vi "Action.vi"() -> ()   [LabVIEW 2014]
uses:
  APIs/Message Queue/WINFAS 2 Message Queue.lvlib
  APIs/Message Queue/Enqueue Message (Array).vi
  APIs/Message Queue/Enqueue Message (Single).vi
  Classes/AutoZero/AutoZero.lvclass
  TypeDefs/STEP State.ctl
  APIs/Message Queue/Message Cluster.ctl
panel:
  in  "CORE":refnum<queue>
  in  "STEP State":T1
  out "AutoZero out":refnum<class "AutoZero.lvclass">
  in  "AutoZero in":refnum<class "AutoZero.lvclass">
  out "error out":errorcluster
  in  "error in (no error)":errorcluster
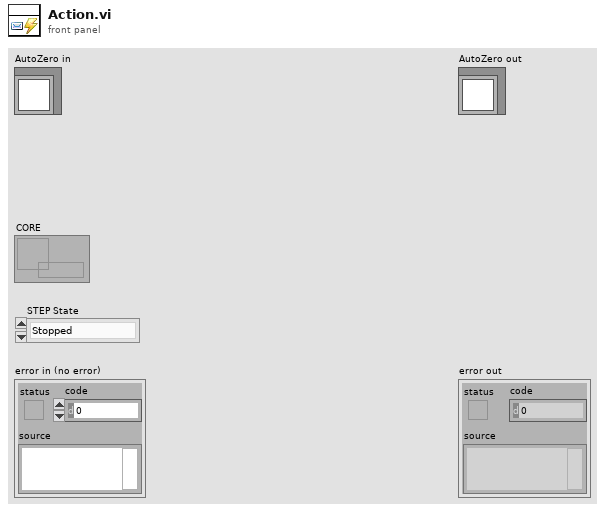
[diagram p1: front panel]
types:
  T1 = typedef "Seq-MathLoop.lvlib/STEP State.ctl" = enum16{"Stopped", "First Call", "Idle...", "Advance OK", "Alarm", "Output Security", "Error"}
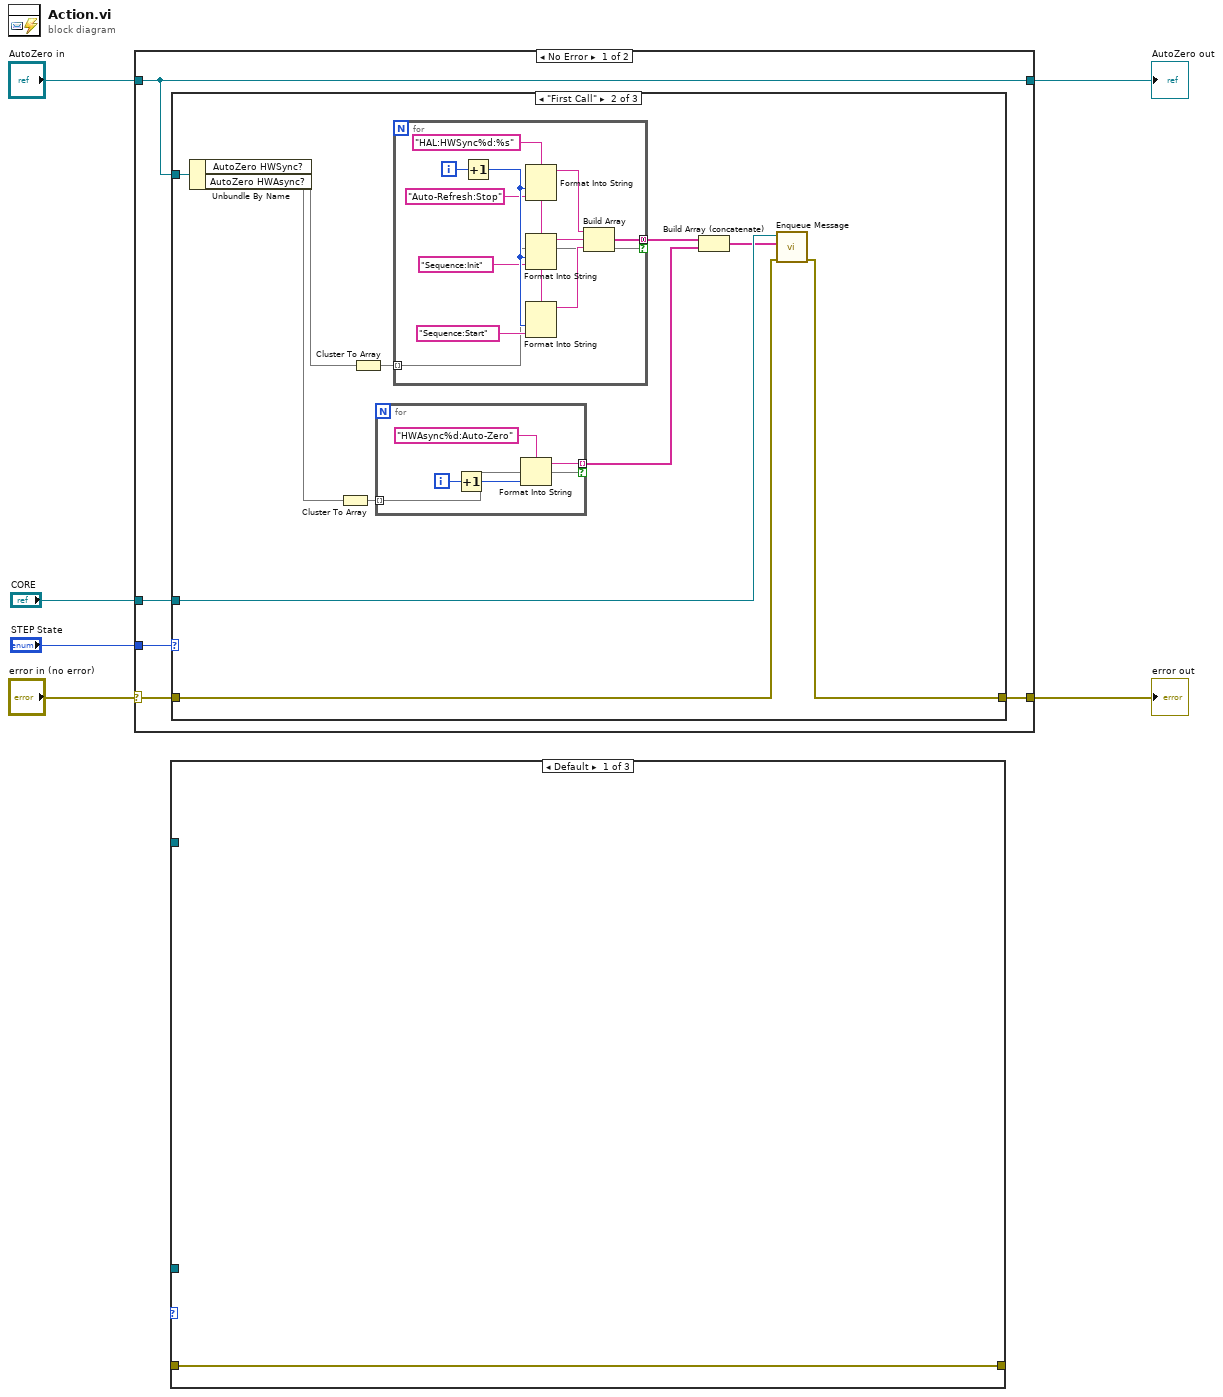
[diagram p0: block diagram]
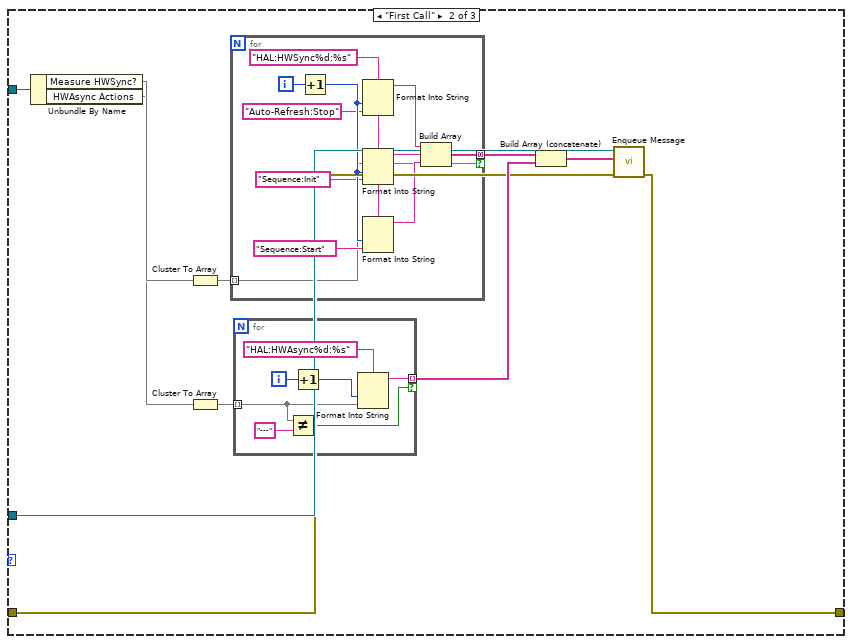
[diagram p2: hidden frame]
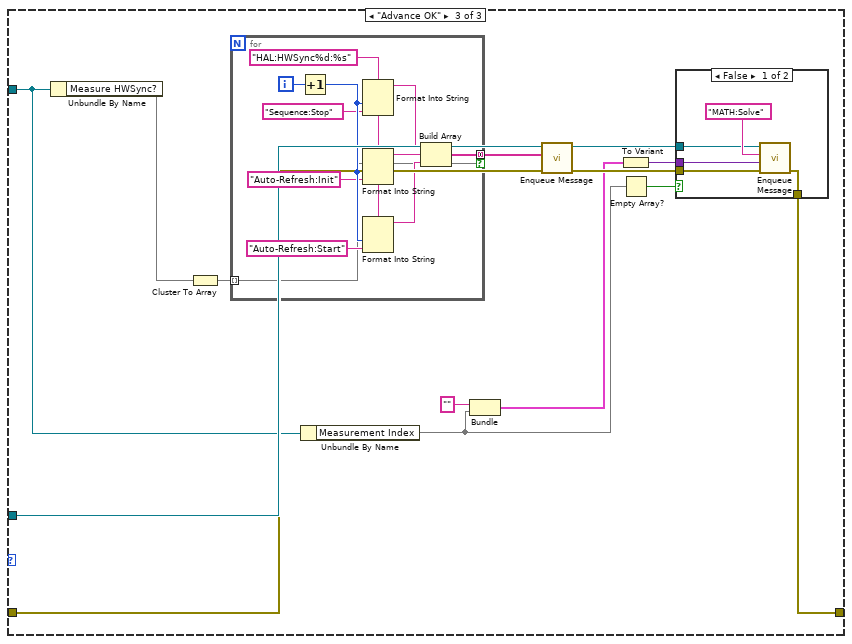
[diagram p3: hidden frame]
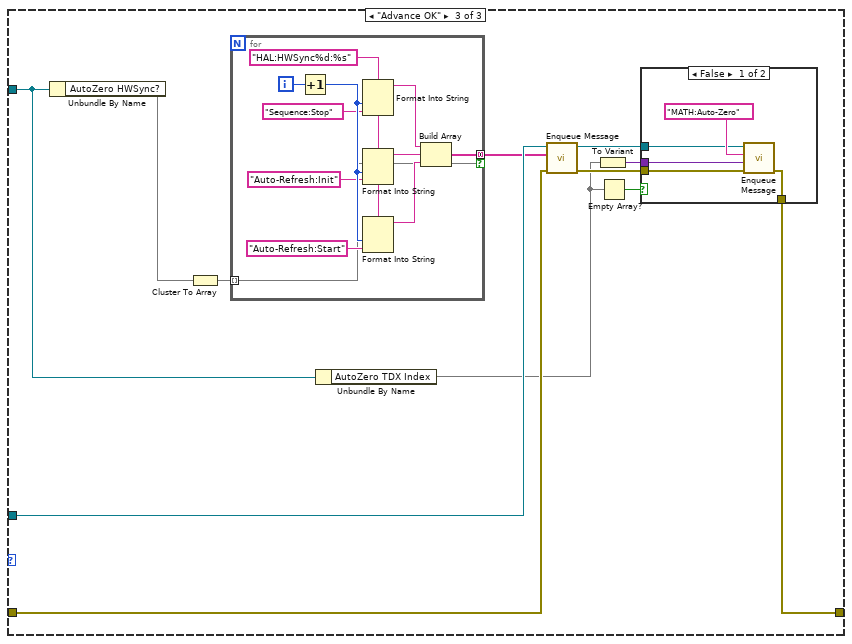
[diagram p6: hidden frame]
diagram:
  n1 = case shown="No Error" "error in (no error)" {
    selector: "error in (no error)" -> [w8 w70]
    tunnel: [w7 w70] -> w3
    tunnel: [w9 w69] -> w5
    tunnel: "AutoZero in" -> [w9 w69]
    tunnel: "CORE" -> [w10 _]
    tunnel: "STEP State" -> [w11 _]
    frame No Error {
      n2 = case shown="\"First Call\"" w11 {
        tunnel: w10 -> [_ w16 w49]
        tunnel: w9 -> [_ w22 w44]
        tunnel: w8 -> [w12 w14 w48]
        tunnel: [w12 w13 w45] -> w7
        frame Default {
        }
        frame "First Call" {
          n3 = Unbundle By Name(w22) -> ("AutoZero HWSync?"=w21, "AutoZero HWAsync?"=w20)
          n4 = Cluster To Array(cluster=w20) -> (array=w19:void[])
          n5 = Cluster To Array(cluster=w21) -> (array=w23:void[])
          n6 = for {
            tunnel: w19 -> [w24] mode=indexing
            tunnel: [w25] -> w17 mode=indexing if=w24
            i -> [w27]
            n7 = Increment(x=w27) -> (x+1=w26:i32)
            n8 = Format Into String(format string="HWAsync%d:Auto-Zero", w26) -> (resulting string=w25:string)  [unwired: 2 in, 1 out]
          }
          n9 = for {
            tunnel: w23 -> [w29] mode=indexing
            tunnel: [w30] -> w18 mode=concatenating if=w29
            i -> [w39]
            w38 = "HAL:HWSync%d:%s" ("format string")
            n10 = Increment(x=w39) -> (x+1=w37:i32)
            n11 = Format Into String(format string=w38, w37, "Auto-Refresh:Stop" ("format string")) -> (resulting string=w33:string)  [unwired: 2 in, 1 out]
            n12 = Format Into String(format string=w38, w37, "Sequence:Init" ("format string")) -> (resulting string=w32:string)  [unwired: 2 in, 1 out]
            n13 = Format Into String(format string=w38, w37, "Sequence:Start" ("format string")) -> (resulting string=w31:string)  [unwired: 2 in, 1 out]
            n14 = Build Array(w33, w32, w31) -> (w30:string[])
          }
          n15 = Build Array (concatenate)(w18, w17) -> (w15:string[])
          n16 = call-poly "Enqueue Message.vi"("error in (no error)"=w14, "Message Array"=w15, "Message Queue"=w16) -> ("error out"=w13:errorcluster)  [unwired: 7 in, 1 out]
        }
        frame "Advance OK" {
          n17 = Unbundle By Name(w44) -> ("AutoZero HWSync?"=w50)
          n18 = Cluster To Array(cluster=w50) -> (array=w51:void[])
          n19 = for {
            tunnel: w51 -> [w58] mode=indexing
            tunnel: [w59] -> w47 mode=concatenating if=w58
            i -> [w68]
            w67 = "HAL:HWSync%d:%s" ("format string")
            n20 = Increment(x=w68) -> (x+1=w66:i32)
            n21 = Format Into String(format string=w67, w66, "Sequence:Stop" ("format string")) -> (resulting string=w62:string)  [unwired: 2 in, 1 out]
            n22 = Format Into String(format string=w67, w66, "Auto-Refresh:Init" ("format string")) -> (resulting string=w61:string)  [unwired: 2 in, 1 out]
            n23 = Format Into String(format string=w67, w66, "Auto-Refresh:Start" ("format string")) -> (resulting string=w60:string)  [unwired: 2 in, 1 out]
            n24 = Build Array(w62, w61, w60) -> (w59:string[])
          }
          n25 = Unbundle By Name(w44) -> ("AutoZero TDX Index"=w41)
          n26 = call-poly "Enqueue Message.vi"("error in (no error)"=w48, "Message Array"=w47, "Message Queue"=w49) -> ("error out"=w46:errorcluster, "dup Message Queue"=w43:refnum<queue>)  [unwired: 7 in]
          n27 = To Variant(anything=w41) -> (Variant=w42:variant)
          n28 = Empty Array?(array=w41) -> (empty?=w40:bool)
          n29 = case shown="False" w40 {
            tunnel: w46 -> [w56 w57]
            tunnel: [w55 w57] -> w45
            tunnel: w43 -> [w53 _]
            tunnel: w42 -> [w52 _]
            frame False {
              n30 = call-poly "Enqueue Message.vi"("error in (no error)"=w56, "Message Data"=w52, "Message"="MATH:Auto-Zero" ("format string"), "Message Queue"=w53) -> ("error out"=w55:errorcluster)  [unwired: 6 in, 1 out]
            }
            frame True {
            }
          }
        }
      }
    }
    frame Error {
    }
  }
  "error out" <- w3
  "AutoZero out" <- w5
  n31 = case shown="Default" {
    selector: _ -> [_ _ _]
    tunnel: _ -> [_ w75 w112]
    tunnel: _ -> [_ w81 w107]
    tunnel: _ -> [w71 w73 w111]
    tunnel: [w71 w72 w108] -> _
    frame Default {
    }
    frame "First Call" {
      n32 = Unbundle By Name(w81) -> ("Measure HWSync?"=w80, "HWAsync Actions"=w79)
      n33 = Cluster To Array(cluster=w80) -> (array=w82:void[])
      n34 = Cluster To Array(cluster=w79) -> (array=w78:void[])
      n35 = for {
        tunnel: w82 -> [w90] mode=indexing
        tunnel: [w91] -> w77 mode=concatenating if=w90
        i -> [w100]
        w99 = "HAL:HWSync%d:%s" ("format string")
        n36 = Increment(x=w100) -> (x+1=w98:i32)
        n37 = Format Into String(format string=w99, w98, "Auto-Refresh:Stop" ("format string")) -> (resulting string=w94:string)  [unwired: 2 in, 1 out]
        n38 = Format Into String(format string=w99, w98, "Sequence:Init" ("format string")) -> (resulting string=w93:string)  [unwired: 2 in, 1 out]
        n39 = Format Into String(format string=w99, w98, "Sequence:Start" ("format string")) -> (resulting string=w92:string)  [unwired: 2 in, 1 out]
        n40 = Build Array(w94, w93, w92) -> (w91:string[])
      }
      n41 = for {
        tunnel: w78 -> [w86] mode=indexing
        tunnel: [w84] -> w76 mode=indexing if=w83
        i -> [w88]
        n42 = Not Equal?(x=w86, y="---") -> (x != y?=w83:bool)
        n43 = Increment(x=w88) -> (x+1=w87:i32)
        n44 = Format Into String(format string="HAL:HWAsync%d:%s", w87, w86) -> (resulting string=w84:string)  [unwired: 2 in, 1 out]
      }
      n45 = Build Array (concatenate)(w77, w76) -> (w74:string[])
      n46 = call-poly "Enqueue Message.vi"("error in (no error)"=w73, "Message Array"=w74, "Message Queue"=w75) -> ("error out"=w72:errorcluster)  [unwired: 7 in, 1 out]
    }
    frame "Advance OK" {
      n47 = Unbundle By Name(w107) -> ("Measure HWSync?"=w113)
      n48 = Cluster To Array(cluster=w113) -> (array=w114:void[])
      n49 = for {
        tunnel: w114 -> [w121] mode=indexing
        tunnel: [w122] -> w110 mode=concatenating if=w121
        i -> [w131]
        w130 = "HAL:HWSync%d:%s" ("format string")
        n50 = Increment(x=w131) -> (x+1=w129:i32)
        n51 = Format Into String(format string=w130, w129, "Sequence:Stop" ("format string")) -> (resulting string=w125:string)  [unwired: 2 in, 1 out]
        n52 = Format Into String(format string=w130, w129, "Auto-Refresh:Init" ("format string")) -> (resulting string=w124:string)  [unwired: 2 in, 1 out]
        n53 = Format Into String(format string=w130, w129, "Auto-Refresh:Start" ("format string")) -> (resulting string=w123:string)  [unwired: 2 in, 1 out]
        n54 = Build Array(w125, w124, w123) -> (w122:string[])
      }
      n55 = Unbundle By Name(w107) -> ("Measurement Index"=w102)
      n56 = Bundle("", "Measurement Index"=w102) -> (w103:cluster{string, "Measurement Index":void})  [unwired: 1 in]
      n57 = call-poly "Enqueue Message.vi"("error in (no error)"=w111, "Message Array"=w110, "Message Queue"=w112) -> ("error out"=w109:errorcluster, "dup Message Queue"=w106:refnum<queue>)  [unwired: 7 in]
      n58 = To Variant(anything=w103) -> (Variant=w105:variant)
      n59 = Empty Array?(array=w102) -> (empty?=w104:bool)
      n60 = case shown="False" w104 {
        tunnel: w109 -> [w119 w120]
        tunnel: [w118 w120] -> w108
        tunnel: w106 -> [w116 _]
        tunnel: w105 -> [w115 _]
        frame False {
          n61 = call-poly "Enqueue Message.vi"("error in (no error)"=w119, "Message Data"=w115, "Message"="MATH:Solve" ("format string"), "Message Queue"=w116) -> ("error out"=w118:errorcluster)  [unwired: 6 in, 1 out]
        }
        frame True {
        }
      }
    }
  }
